vi "Tube Avg Sound Speed.vi"(4 "Atm. Pressure (pascals)":dbl=101325.0, 6 "Humidity (%)":dbl=60.0 format="%_4g", 8 "Error In":errorcluster, 10 "Range":dbl, 11 "All Temps":dbl[](array[numeric])) -> (0 "Error Out":errorcluster, 2 "Cramer Speed of Sound in Tube Length at Tc":dbl, 3 "Speed of Sound in Tube Length at Tc":dbl)   [LabVIEW 2014, in "Analysis.lvlib"]
uses:
  Analysis.lvlib
  <vilib>/Analysis/baseanly.llb/Mean (DBL).vi
  <vilib>/Analysis/NI_AALBase.lvlib
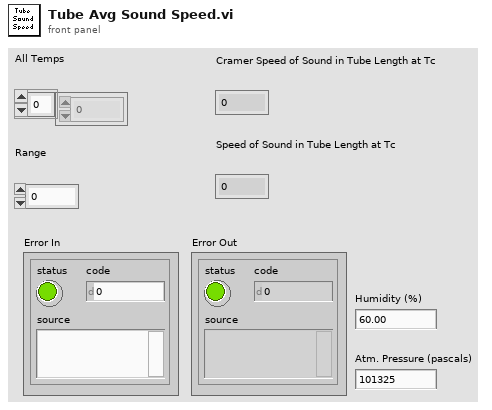
[diagram p1: front panel]
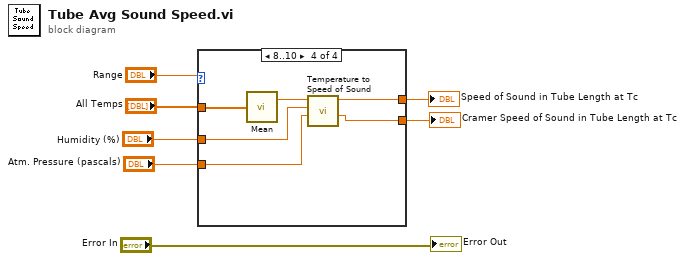
[diagram p0: block diagram]
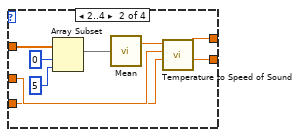
[diagram p3: hidden frame]
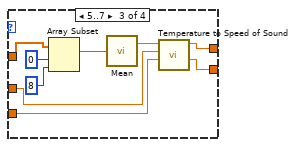
[diagram p4: hidden frame]
diagram:
  n1 = case shown="8..10" "Range" {
    tunnel: "All Temps" -> [_ w16 w21 w30]
    tunnel: [_ w11 w20 w29] -> w5
    tunnel: [_ w10 w19 w28] -> w3
    tunnel: "Humidity (%)" -> [_ w9 w18 w27]
    tunnel: "Atm. Pressure (pascals)" -> [_ w8 w17 w26]
    frame 0, Default {
    }
    frame 2..4 {
      n2 = Array Subset(array=w16, index=0, length=5) -> (w13:dbl[])
      n3 = call-poly <vilib>:"Mean.vi"("X"=w13) -> ("mean"=w12:dbl)  [unwired: 1 out]
      n4 = call "Temperature to Speed of Sound.vi"("Pressure (pascals)"=w8, "Humidity"=w9, "Temperature"=w12) -> ("Cramer Speed of Sound at Tc Humid Air (m/s)"=w10:dbl, "Speed of Sound at Tc Dry Air (m/s)"=w11:dbl)  [unwired: 7 in]
    }
    frame 5..7 {
      n5 = Array Subset(array=w21, index=0, length=8) -> (w23:dbl[])
      n6 = call-poly <vilib>:"Mean.vi"("X"=w23) -> ("mean"=w22:dbl)  [unwired: 1 out]
      n7 = call "Temperature to Speed of Sound.vi"("Pressure (pascals)"=w17, "Humidity"=w18, "Temperature"=w22) -> ("Cramer Speed of Sound at Tc Humid Air (m/s)"=w19:dbl, "Speed of Sound at Tc Dry Air (m/s)"=w20:dbl)  [unwired: 7 in]
    }
    frame 8..10 {
      n8 = call-poly <vilib>:"Mean.vi"("X"=w30) -> ("mean"=w31:dbl)  [unwired: 1 out]
      n9 = call "Temperature to Speed of Sound.vi"("Pressure (pascals)"=w26, "Humidity"=w27, "Temperature"=w31) -> ("Cramer Speed of Sound at Tc Humid Air (m/s)"=w28:dbl, "Speed of Sound at Tc Dry Air (m/s)"=w29:dbl)  [unwired: 7 in]
    }
  }
  "Speed of Sound in Tube Length at Tc" <- w5
  "Cramer Speed of Sound in Tube Length at Tc" <- w3
  "Error Out" <- "Error In"
